vi "Remove Script.vi"(8 "error in":errorcluster, 10 "Script UI Ctrl Ref":T2, 11 "Script Meas Config Ctrl Ref":T1) -> (0 "error out":errorcluster)   [LabVIEW 2025, in "Fgen Script Mode UI.lvlib"]
uses:
  Fgen Script Mode UI.lvlib
  Typedef/Script Meas Config Ctrl Ref.ctl
  Typedef/Script UI Ctrl Ref.ctl
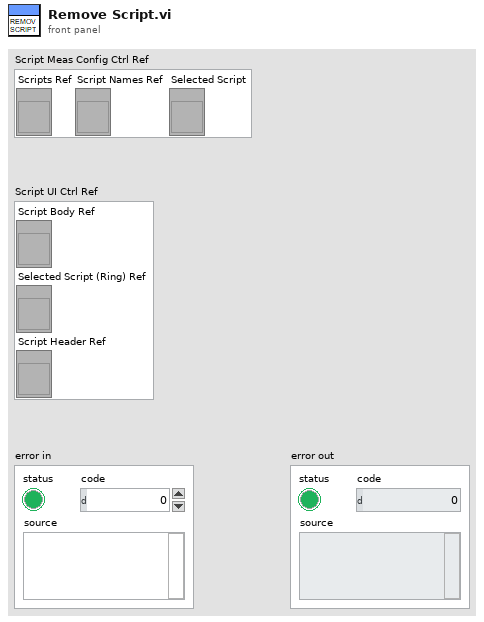
[diagram p1: front panel]
types:
  T1 = typedef "Fgen Script Mode UI.lvlib/Script Meas Config Ctrl Ref.ctl" = cluster{"Scripts Ref":refnum<vi>, "Script Names Ref":refnum<vi>, "Selected Script":refnum<vi>}
  T2 = typedef "Fgen Script Mode UI.lvlib/Script UI Ctrl Ref.ctl" = cluster{"Script Body Ref":refnum<vi>, "Selected Script (Ring) Ref":refnum<vi>, "Script Header Ref":refnum<vi>}
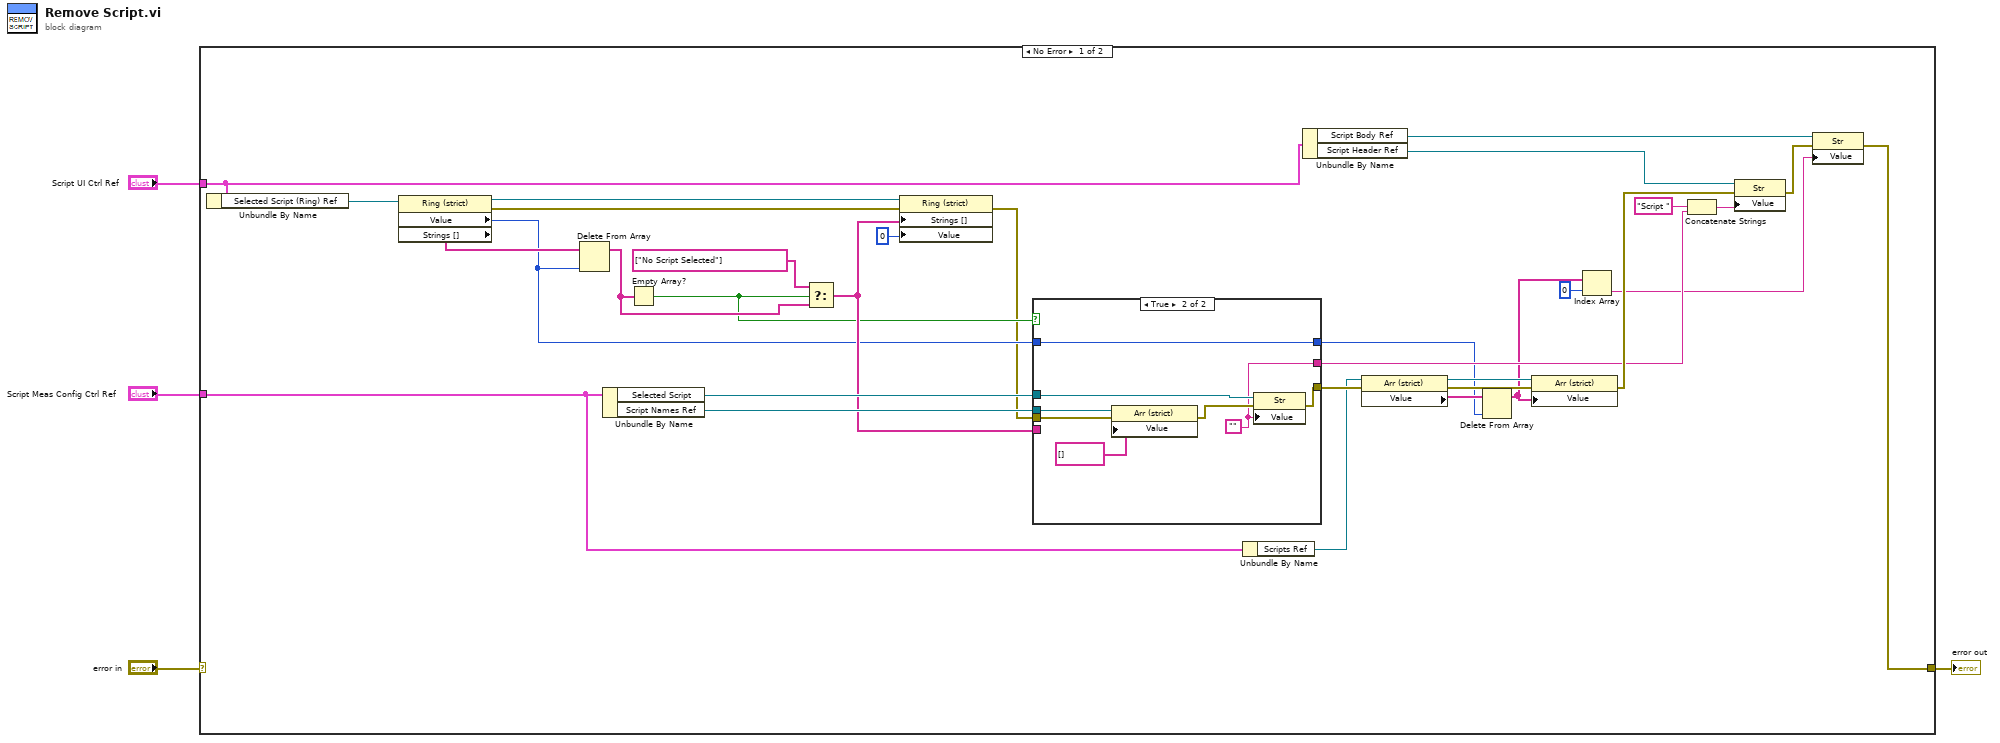
[diagram p0: block diagram]
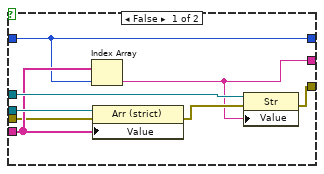
[diagram p2: hidden frame]
diagram:
  n1 = case shown="No Error" "error in" {
    selector: "error in" -> [_ w53]
    tunnel: [w36 w53] -> w3
    tunnel: "Script Meas Config Ctrl Ref" -> [w6 _]
    tunnel: "Script UI Ctrl Ref" -> [w35 _]
    frame No Error {
      n2 = Unbundle By Name(w35) -> ("Selected Script (Ring) Ref"=w34:refnum<vi>)
      n3 = property class="Ring (strict)"(reference=w34) -> (reference out=w20:refnum<vi>, error out=w19:errorcluster, "Value"=w12:u16, "Strings []"=w21:string[])  [unwired: 1 in]
      n4 = Delete From Array(array=w21, index=w12) -> (array with subset deleted=w18:string[])  [unwired: 1 in, 1 out]
      n5 = Unbundle By Name(w6) -> ("Selected Script"=w26:refnum<vi>, "Script Names Ref"=w27:refnum<vi>)
      n6 = Empty Array?(array=w18) -> (empty?=w14:bool)
      n7 = Select(t=string[] ["No Script Selected"] ("Strings []"), s=w14, f=w18) -> (s? t:f=w16:string[])
      n8 = property class="Ring (strict)"(reference=w20, error in=w19, "Strings []"=w16, "Value"=u16 0) -> (error out=w7:errorcluster)  [unwired: 1 out]
      n9 = case shown="True" w14 {
        tunnel: w27 -> [w44 w52]
        tunnel: w26 -> [w43 w51]
        tunnel: [w41 w49] -> w25
        tunnel: w16 -> [w40 _]
        tunnel: w12 -> [w38 w46]
        tunnel: [w39 w47] -> w13
        tunnel: [w38 w46] -> w11
        tunnel: w7 -> [w37 w45]
        frame False {
          n10 = Index Array(array=w40, index=w38) -> (element=w39:string)
          n11 = property class="Arr (strict)"(reference=w44, error in=w37, "Value"=w40) -> (error out=w42:errorcluster)  [unwired: 1 out]
          n12 = property class="Str"(reference=w43, error in=w42, "Value"=w39) -> (error out=w41:errorcluster)  [unwired: 1 out]
        }
        frame True {
          w47 = ""
          n13 = property class="Arr (strict)"(reference=w52, error in=w45, "Value"=string[] []) -> (error out=w50:errorcluster)  [unwired: 1 out]
          n14 = property class="Str"(reference=w51, error in=w50, "Value"=w47) -> (error out=w49:errorcluster)  [unwired: 1 out]
        }
      }
      n15 = Unbundle By Name(w6) -> ("Scripts Ref"=w5:refnum<vi>)
      n16 = Unbundle By Name(w35) -> ("Script Body Ref"=w30:refnum<vi>, "Script Header Ref"=w33:refnum<vi>)
      n17 = property class="Arr (strict)"(reference=w5, error in=w25) -> (reference out=w29:refnum<vi>, error out=w24:errorcluster, "Value"=w28:string[])
      n18 = Delete From Array(array=w28, index=w11) -> (array with subset deleted=w10:string[])  [unwired: 1 in, 1 out]
      n19 = property class="Arr (strict)"(reference=w29, error in=w24, "Value"=w10) -> (error out=w23:errorcluster)  [unwired: 1 out]
      n20 = Index Array(array=w10, index=0) -> (element=w8:string)
      n21 = Concatenate Strings("Script " ("format string"), w13) -> (w31:string)
      n22 = property class="Str"(reference=w33, error in=w23, "Value"=w31) -> (error out=w22:errorcluster)  [unwired: 1 out]
      n23 = property class="Str"(reference=w30, error in=w22, "Value"=w8) -> (error out=w36:errorcluster)  [unwired: 1 out]
    }
    frame Error {
    }
  }
  "error out" <- w3
